vi "Begin.vi"(8 "error in":errorcluster) -> (0 "error out":errorcluster)   [LabVIEW 2016]
doc: "Called before other user functions, this VI is expected to open initial I/O refnums, load in file data, and do all program initialization. Notice that the <B>error out</B> terminal is simply used for data flow. Wiring it to other structures or subVIs ensures that this VI runs first."
uses:
  <vilib>/Rock Robotics/SystemInterfaces/DIO/FPGA_DIOPWMChannel.ctl
  <vilib>/Rock Robotics/WPI/SafetyOutput/WPI_SafetyOutputConfigMenu.ctl
  <vilib>/Rock Robotics/WPI/DriverStation/WPI_DriverStationRobotMode2.ctl
  <vilib>/Rock Robotics/WPI/Joystick/WPI_JoystickDeviceEnum.ctl
  <vilib>/Rock Robotics/SystemInterfaces/DIO/FPGA_DIOChannel.ctl
  <vilib>/Rock Robotics/WPI/Encoder/WPI_EncoderType.ctl
  NI WPI/WPI_SerialPort_USB.ctl
  <vilib>/Rock Robotics/WPI/ThirdParty/CanMotor/TalonSRX/WPI_CANTalonSRX_APIControlMode.ctl
  <vilib>/Rock Robotics/WPI/Solenoid/WPI_SolenoidChannel.ctl
  <vilib>/Rock Robotics/SystemInterfaces/i2clib/i2c_bus.ctl
  Robot Global Data.vi
  <vilib>/Rock Robotics/Network Tables/NT Write String Array.vi
  <vilib>/Rock Robotics/WPI/Counter/WPI_CounterDigitalInputToDigitalSource.vi
  navX Library v2/IO/Open/Z900_navX_Open_Serial.vi
  <vilib>/Rock Robotics/WPI/Solenoid/WPI_SolenoidOpenSingle.vi
  <vilib>/Rock Robotics/WPI/MotorControl/WPI_MotorControlOpen VictorSP.vi
  <vilib>/Rock Robotics/WPI/RobotDrive/WPI_RobotDriveOpen4MotorWithVictorSP.vi
  navX Library v2/navX Library v2.lvlib
  NI WPI/NI WPI Serial USB.lvlib
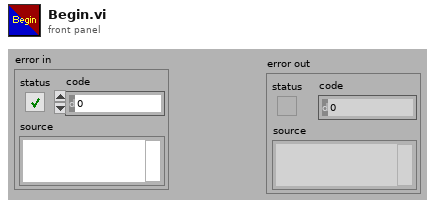
[diagram p1: front panel]
types:
  T1 = typedef "i2c_bus.ctl" = enum16{"I2C On-Board", "I2C MXP", "Invalid"}
  T2 = typedef "WPI_SolenoidChannel.ctl" = enum8{"Solenoid 0", "Solenoid 1", "Solenoid 2", "Solenoid 3", "Solenoid 4", "Solenoid 5", "Solenoid 6", "Solenoid 7", "Invalid"}
  T3 = typedef "FPGA_DIOPWMChannel.ctl" = enum8{"PWM 0", "PWM 1", "PWM 2", "PWM 3", "PWM 4", "PWM 5", "PWM 6", "PWM 7", "PWM 8", "PWM 9", "PWM MXP 0", "PWM MXP 1", "PWM MXP 2", "PWM MXP 3", "PWM MXP 4", "PWM MXP 5", "PWM MXP 6", "PWM MXP 7", "PWM MXP 8", "PWM MXP 9", "Invalid"}
  T4 = typedef "WPI_JoystickDeviceEnum.ctl" = enum16{"USB 0", "USB 1", "USB 2", "USB 3", "USB 4", "USB 5"}
  T5 = typedef "WPI_CANTalonSRX_APIControlMode.ctl" = enum8{"Percent VBus", "Speed", "Position", "Slave", "Unchanged / Invalid", "Voltage Compensation", "Current", "Motion Profile", "Motion Magic"}
  T6 = typedef "NI WPI Serial USB.lvlib/WPI_SerialPort_USB.ctl" = enum16{"Onboard RS-232", "MXP TTL", "USB"}
  T7 = typedef "WPI_EncoderType.ctl" = enum16{"1x", "2x", "4x"}
  T8 = typedef "FPGA_DIOChannel.ctl" = enum8{"DIO 0", "DIO 1", "DIO 2", "DIO 3", "DIO 4", "DIO 5", "DIO 6", "DIO 7", "DIO 8", "DIO 9", "DIO MXP 0", "DIO MXP 1", "DIO MXP 2", "DIO MXP 3", "DIO MXP 4", "DIO MXP 5", "DIO MXP 6", "DIO MXP 7", "DIO MXP 8", "DIO MXP 9", "DIO MXP 10", "DIO MXP 11", "DIO MXP 12", "DIO MXP 13", "DIO MXP 14", "DIO MXP 15", "SPI Port CS1", "SPI Port CS2", "SPI Port CS3", "SPI Port MISO", "SPI Port MOSI", "Invalid"}
  T9 = typedef "WPI_DriverStationRobotMode2.ctl" = enum16{"Autonomous Disabled", "Autonomous Enabled", "Teleop Disabled", "Teleop Enabled", "Disconnected", "Finish", "Test Disabled", "Test Enabled", "Emergency Stopped"}
  T10 = typedef "WPI_SafetyOutputConfigMenu.ctl" = enum16{"Enable", "Disable"}
  T11 = typedef "WPI_JoystickDevRef.ctl" = cluster{"Device":T4}
  T12 = typedef "WPI_I2CDevRef.ctl" = cluster{"DevStatus":errorcluster, "Device Address":u8, "Handle":i32, "I2C Bus":T1}
  T13 = typedef "WPI_MotorControlDeviceRef.ctl" = cluster{"DeviceStatus":errorcluster, "Type":T14, "PWM":cluster{"PWM Channel":T3, "DeadBand":T15}, "CAN":cluster{"Device Number":u8, "SetOutput VI Ref":variant, "GetOutput VI Ref":variant, "Enable VI Ref":variant, "Disable VI Ref":variant, "Data":variant}, "Invert":bool}
  T14 = typedef "WPI_MotorControlType.ctl" = enum16{"PWM", "CAN"}
  T15 = typedef "WPI_PWMDeadband.ctl" = cluster{"Name":string, "maxPositivePwm":i32, "minPositivePwm":i32, "centerPwm":i32, "maxNegativePwm":i32, "minNegativePwm":i32, "angularRange":u16}
  T16 = typedef "WPI_RobotDriveDevRef.ctl" = cluster{"DevStatus":errorcluster, "Motors[]":T13[], "Square Inputs":bool, "Max Output":dbl}
  T17 = typedef "WPI_DigitalInputDevRef.ctl" = cluster{"DevStatus":errorcluster, "DIO Channel":T8}
  T18 = typedef "FPGA_CounterEncoderSourceConvertionLVSourceType.ctl" = cluster{"DevStatus":errorcluster, "AnalogTriggerMode?":bool, "DigitalMode":cluster{"DIO Channel":T19}, "AnalogTriggerMode":cluster{"AnalogTriggerIndex":T20, "OutputType":T21}}
  T19 = typedef "FPGA_DIODigitalSourceChannel.ctl" = enum8{"DIO 0", "DIO 1", "DIO 2", "DIO 3", "DIO 4", "DIO 5", "DIO 6", "DIO 7", "DIO 8", "DIO 9", "DIO MXP 0", "DIO MXP 1", "DIO MXP 2", "DIO MXP 3", "DIO MXP 4", "DIO MXP 5", "DIO MXP 6", "DIO MXP 7", "DIO MXP 8", "DIO MXP 9", "DIO MXP 10", "DIO MXP 11", "DIO MXP 12", "DIO MXP 13", "DIO MXP 14", "DIO MXP 15", "Disabled"}
  T20 = typedef "FPGA_AnalogTriggerIndex.ctl" = enum8{"Trig 0", "Trig 1", "Trig 2", "Trig 3", "Trig 4", "Trig 5", "Trig 6", "Trig 7", "Invalid"}
  T21 = typedef "FPGA_AnalogTriggerOutType.ctl" = enum16{"InWindow", "TriggerState", "Rising", "Falling"}
  T22 = typedef "WPI_EncoderDevRef.ctl" = cluster{"DevStatus":errorcluster, "EncoderIndex":T23, "CounterIndex":T24, "DistancePerCount":dbl, "Decoding Type":T7}
  T23 = typedef "FPGA_EncoderIdx.ctl" = enum8{"Enc 0", "Enc 1", "Enc 2", "Enc 3", "Enc 4", "Enc 5", "Enc 6", "Enc 7", "Invalid"}
  T24 = typedef "FPGA_CounterCtrSystemIndex.ctl" = enum8{"Ctr 0", "Ctr 1", "Ctr 2", "Ctr 3", "Ctr 4", "Ctr 5", "Ctr 6", "Ctr 7", "Invalid"}
  T25 = typedef "navX Library v2.lvlib/Z900_navX_DeviceTypeDef.ctl" = cluster{"Interface":cluster{"Protocol":T26, "Update Rate (4Hz-100Hz)":u8, "navX Open TypeDef":variant}, "Notify Packet":refnum<notifier>, "Loop VI Refnum":refnum<vi>, "Ready to Close Occurrence Refnum":refnum<k4>}
  T26 = typedef "navX Library v2.lvlib/Z900_navX_ProtocolTypeDef.ctl" = enum16{"SERIAL", "I2C", "SPI"}
  T27 = typedef "WPI_SolenoidDevRef.ctl" = cluster{"DevStatus":errorcluster, "Pneumatics Control Module":u8, "Forward Solenoid Channel":T2, "Reverse Solenoid Channel":T2}
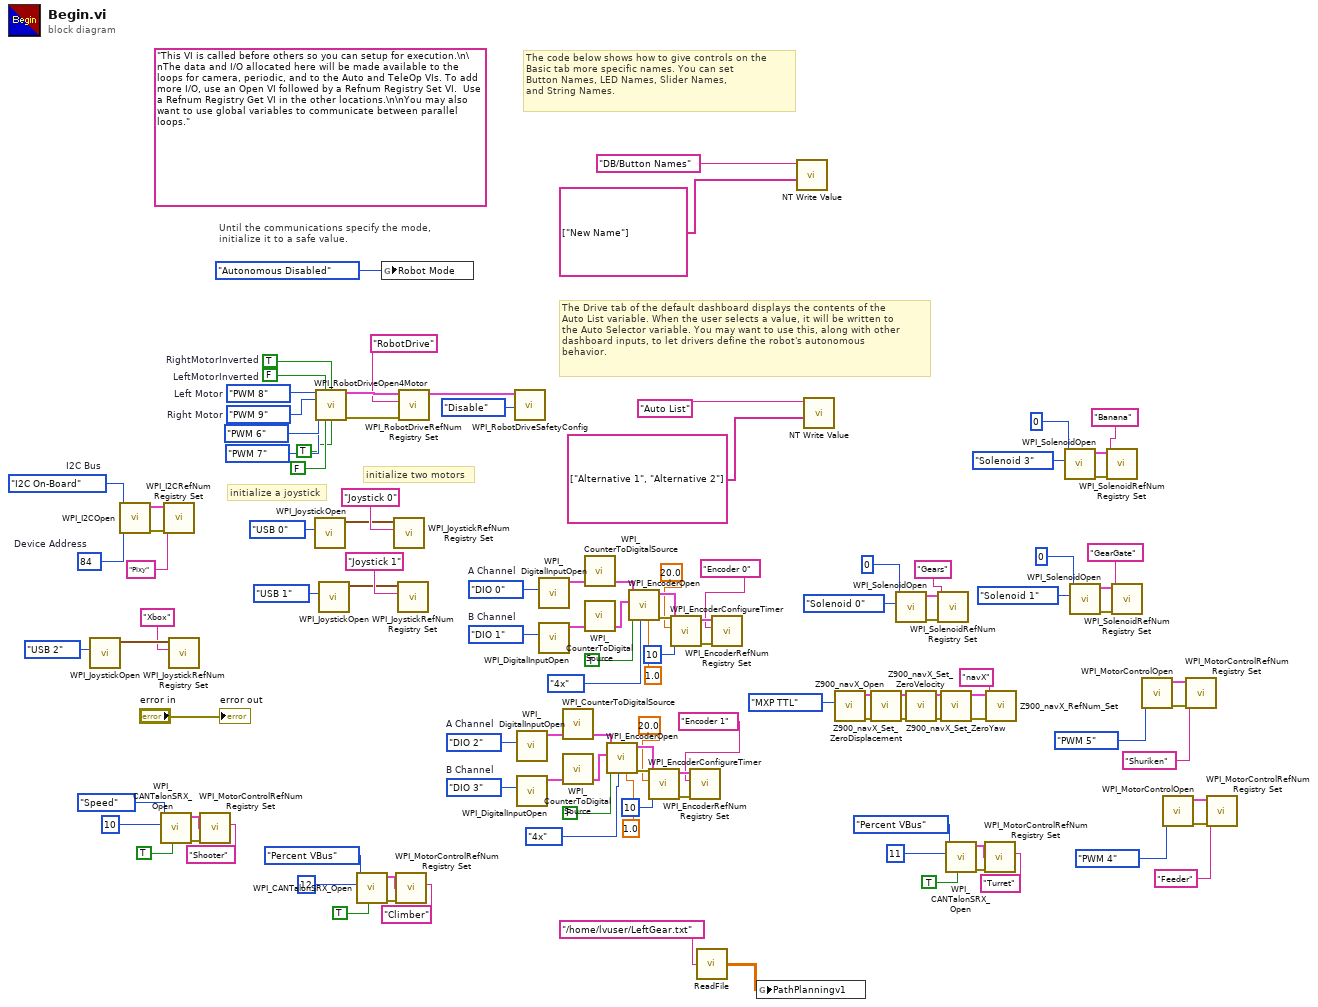
[diagram p0: block diagram]
diagram:
  w8 = u8 84  # Device Address
  w9 = i2c_bus."I2C On-Board"  # I2C Bus
  w81 = FPGA_DIOChannel."DIO 3"  # B Channel
  w80 = FPGA_DIOChannel."DIO 2"  # A Channel
  w97 = FPGA_DIOChannel."DIO 1"  # B Channel
  w96 = FPGA_DIOChannel."DIO 0"  # A Channel
  (unwired) "This VI is called before others so you can setup for execution.\n\nThe data and I/O allocated here will be made available to the loops for camera, periodic, and to the Auto and TeleOp VIs. To add more I/O, use an Open VI followed by a Refnum Registry Set VI.  Use a Refnum Registry Get VI in the other locations.\n\nYou may also want to use global variables to communicate between parallel loops."
  w112 = FPGA_DIOPWMChannel."PWM 9"  # Right Motor
  w113 = FPGA_DIOPWMChannel."PWM 8"  # Left Motor
  w117 = FALSE  # LeftMotorInverted
  w118 = TRUE  # RightMotorInverted
  # "The Drive tab of the default dashboard displays the contents of the\nAuto List variable. When the user selects a value, it will be written to\nthe Auto Selector variable. You may want to use this, along with other\ndashboard inputs, to let drivers define the robot's autonomous\nbehavior."
  # "The code below shows how to give controls on the\nBasic tab more specific names. You can set\nButton Names, LED Names, Slider Names,\nand String Names."
  # "initialize a joystick"
  # "Until the communications specify the mode,\ninitialize it to a safe value."
  # "initialize two motors"
  n1 = call <vilib>:"WPI_JoystickOpen.vi"("JoystickDevice"=WPI_JoystickDeviceEnum."USB 2") -> ("JoystickDevRef"=w21:T11)  [unwired: 10 in]
  n2 = call <vilib>:"WPI_I2COpen.vi"("Device Address"=w8, "I2C Bus"=w9) -> ("error out"=w7:errorcluster, "I2CDevRef"=w6:T12)  [unwired: 8 in]
  n3 = call <vilib>:"WPI_CANTalonSRX_Open.vi"("Invert"=TRUE, "Device Number"=10, "Control Mode"=WPI_CANTalonSRX_APIControlMode."Speed") -> ("error out"=w48:errorcluster, "CAN Talon SRX Ref"=w49:T13)  [unwired: 7 in]
  n4 = call <vilib>:"WPI_I2CRefNum Registry Set.vi"("error in (no error)"=w7, "refnum name"="Pixy", "I2CDevRef"=w6) -> ()  [unwired: 7 in, 2 out]
  n5 = call <vilib>:"WPI_JoystickRefNum Registry Set.vi"("refnum name"="Xbox", "JoystickDevRef"=w21) -> ()  [unwired: 8 in, 2 out]
  n6 = call <vilib>:"WPI_MotorControlRefNum Registry Set.vi"("error in (no error)"=w48, "refnum name"="Shooter", "MotorControlDevRef"=w49) -> ()  [unwired: 7 in, 2 out]
  n7 = call <vilib>:"WPI_JoystickOpen.vi"("JoystickDevice"=WPI_JoystickDeviceEnum."USB 0") -> ("JoystickDevRef"=w107:T11)  [unwired: 10 in]
  n8 = call-poly <vilib>:"WPI_RobotDriveOpen4Motor.vi"("Rear Left Motor"=w113, "Rear Left Motor Inverted"=w117, "Rear Right Motor Inverted"=w118, "Rear Right Motor"=w112, "Front Left Motor"=FPGA_DIOPWMChannel."PWM 6", "Front Right Motor"=FPGA_DIOPWMChannel."PWM 7", "Front Left Motor Inverted"=FALSE, "Front Right Motor Inverted"=TRUE) -> ("RobotDriveDevRef"=w116:T16, "error out"=w114:errorcluster)  [unwired: 6 in]
  n9 = call <vilib>:"WPI_JoystickOpen.vi"("JoystickDevice"=WPI_JoystickDeviceEnum."USB 1") -> ("JoystickDevRef"=w99:T11)  [unwired: 10 in]
  n10 = call <vilib>:"WPI_CANTalonSRX_Open.vi"("Invert"=TRUE, "Device Number"=12, "Control Mode"=WPI_CANTalonSRX_APIControlMode."Percent VBus") -> ("error out"=w42:errorcluster, "CAN Talon SRX Ref"=w43:T13)  [unwired: 7 in]
  n11 = global write "Robot Global Data.vi" "Robot Mode"(WPI_DriverStationRobotMode2."Autonomous Disabled" ("Robot Mode")) -> ()
  n12 = call <vilib>:"WPI_JoystickRefNum Registry Set.vi"("refnum name"="Joystick 0", "JoystickDevRef"=w107) -> ()  [unwired: 8 in, 2 out]
  n13 = call <vilib>:"WPI_MotorControlRefNum Registry Set.vi"("error in (no error)"=w42, "refnum name"="Climber", "MotorControlDevRef"=w43) -> ()  [unwired: 7 in, 2 out]
  n14 = call <vilib>:"WPI_JoystickRefNum Registry Set.vi"("refnum name"="Joystick 1", "JoystickDevRef"=w99) -> ()  [unwired: 8 in, 2 out]
  n15 = call <vilib>:"WPI_RobotDriveRefNum Registry Set.vi"("error in (no error)"=w114, "refnum name"="RobotDrive", "RobotDriveDevRef"=w116) -> ("RobotDriveDevRef"=w111:T16)  [unwired: 1 in, 7 out]
  n16 = call <vilib>:"WPI_RobotDriveSafetyConfig.vi"("mode"=WPI_SafetyOutputConfigMenu."Disable", "RobotDriveDevRef"=w111) -> ()  [unwired: 8 in, 2 out]
  n17 = call <vilib>:"WPI_DigitalInputOpen.vi"("DIO Channel"=w80) -> ("DigitalInputDevRef"=w77:T17)  [unwired: 1 in, 9 out]
  n18 = call <vilib>:"WPI_DigitalInputOpen.vi"("DIO Channel"=w81) -> ("DigitalInputDevRef"=w78:T17)  [unwired: 1 in, 9 out]
  n19 = call <vilib>:"WPI_DigitalInputOpen.vi"("DIO Channel"=w96) -> ("DigitalInputDevRef"=w93:T17)  [unwired: 1 in, 9 out]
  n20 = call <vilib>:"WPI_DigitalInputOpen.vi"("DIO Channel"=w97) -> ("DigitalInputDevRef"=w94:T17)  [unwired: 1 in, 9 out]
  n21 = call-poly <vilib>:"WPI_CounterToDigitalSource.vi"("DigitalInputDevRef"=w77) -> ("Digital Source"=w76:T18)  [unwired: 6 out]
  n22 = call-poly <vilib>:"WPI_CounterToDigitalSource.vi"("DigitalInputDevRef"=w78) -> ("Digital Source"=w79:T18)  [unwired: 6 out]
  n23 = call-poly <vilib>:"WPI_CounterToDigitalSource.vi"("DigitalInputDevRef"=w93) -> ("Digital Source"=w92:T18)  [unwired: 6 out]
  n24 = call-poly <vilib>:"WPI_CounterToDigitalSource.vi"("DigitalInputDevRef"=w94) -> ("Digital Source"=w95:T18)  [unwired: 6 out]
  n25 = call <vilib>:"WPI_EncoderOpen.vi"("DistancePerCount"=1.0, "Decoding Type"=WPI_EncoderType."4x", "Invert Direction (False)"=FALSE, "BSource"=w79, "ASource"=w76) -> ("error out"=w74:errorcluster, "EncoderDevRef"=w73:T22)  [unwired: 3 in, 2 out]
  n26 = call <vilib>:"WPI_EncoderOpen.vi"("DistancePerCount"=1.0, "Decoding Type"=WPI_EncoderType."4x", "Invert Direction (False)"=TRUE, "BSource"=w95, "ASource"=w92) -> ("error out"=w88:errorcluster, "EncoderDevRef"=w87:T22)  [unwired: 3 in, 2 out]
  n27 = call <vilib>:"WPI_EncoderConfigureTimer.vi"("error in (no error)"=w74, "Number Samples to Average"=u8 10, "Minimum Rate"=20.0, "EncoderDevRef"=w73) -> ("error out"=w70:errorcluster, "EncoderDevRef"=w69:T22)  [unwired: 6 in]
  n28 = call <vilib>:"WPI_EncoderConfigureTimer.vi"("error in (no error)"=w88, "Number Samples to Average"=u8 10, "Minimum Rate"=20.0, "EncoderDevRef"=w87) -> ("error out"=w84:errorcluster, "EncoderDevRef"=w83:T22)  [unwired: 6 in]
  n29 = call <vilib>:"WPI_EncoderRefNum Registry Set.vi"("error in (no error)"=w70, "refnum name"="Encoder 1", "EncoderDevRef"=w69) -> ()  [unwired: 7 in, 2 out]
  n30 = call "ReadFile.vi"("Name"="/home/lvuser/LeftGear.txt") -> ("Array - Numeric"=w3:dbl[][])
  n31 = call <vilib>:"WPI_EncoderRefNum Registry Set.vi"("error in (no error)"=w84, "refnum name"="Encoder 0", "EncoderDevRef"=w83) -> ()  [unwired: 7 in, 2 out]
  n32 = global write "Robot Global Data.vi" "PathPlanningv1"(w3) -> ()
  n33 = call-poly <vilib>:"NT Write Value.vi"("String Array"=string[] ["New Name"], "Name"="DB/Button Names") -> ()  [unwired: 9 in, 1 out]
  n34 = call-poly <vilib>:"NT Write Value.vi"("String Array"=string[] ["Alternative 1", "Alternative 2"], "Name"="Auto List") -> ()  [unwired: 9 in, 1 out]
  n35 = call-poly "Z900_navX_Open.vi"("Serial Port"=WPI_SerialPort_USB."MXP TTL") -> ("error out"=w56:errorcluster, "navX Device"=w61:T25)  [unwired: 9 in]
  n36 = call "Z900_navX_Set_ZeroDisplacement.vi"("error in (no error)"=w56, "navX Device"=w61) -> ("error out"=w55:errorcluster, "navX Device"=w60:T25)  [unwired: 8 in]
  n37 = call-poly <vilib>:"WPI_SolenoidOpen.vi"("Solenoid Channel"=WPI_SolenoidChannel."Solenoid 0", "Pneumatics Control Module (0)"=u8 0) -> ("error out"=w41:errorcluster, "SolenoidDevRef"=w40:T27)  [unwired: 8 in]
  n38 = call "Z900_navX_Set_ZeroVelocity.vi"("error in (no error)"=w55, "navX Device"=w60) -> ("error out"=w54:errorcluster, "navX Device"=w59:T25)  [unwired: 8 in]
  n39 = call <vilib>:"WPI_SolenoidRefNum Registry Set.vi"("error in (no error)"=w41, "refnum name"="Gears", "SolenoidDevRef"=w40) -> ()  [unwired: 7 in, 2 out]
  n40 = call "Z900_navX_Set_ZeroYaw.vi"("error in (no error)"=w54, "navX Device"=w59) -> ("error out"=w57:errorcluster, "navX Device"=w58:T25)  [unwired: 8 in]
  n41 = call <vilib>:"WPI_CANTalonSRX_Open.vi"("Invert"=TRUE, "Device Number"=11, "Control Mode"=WPI_CANTalonSRX_APIControlMode."Percent VBus") -> ("error out"=w31:errorcluster, "CAN Talon SRX Ref"=w32:T13)  [unwired: 7 in]
  n42 = call <vilib>:"WPI_MotorControlRefNum Registry Set.vi"("error in (no error)"=w31, "refnum name"="Turret", "MotorControlDevRef"=w32) -> ()  [unwired: 7 in, 2 out]
  n43 = call "Z900_navX_RefNum_Set.vi"("error in (no error)"=w57, "refnum name"="navX", "navX Device"=w58) -> ()  [unwired: 7 in, 2 out]
  n44 = call-poly <vilib>:"WPI_SolenoidOpen.vi"("Solenoid Channel"=WPI_SolenoidChannel."Solenoid 3", "Pneumatics Control Module (0)"=u8 0) -> ("error out"=w14:errorcluster, "SolenoidDevRef"=w13:T27)  [unwired: 8 in]
  n45 = call-poly <vilib>:"WPI_SolenoidOpen.vi"("Solenoid Channel"=WPI_SolenoidChannel."Solenoid 1", "Pneumatics Control Module (0)"=u8 0) -> ("error out"=w26:errorcluster, "SolenoidDevRef"=w25:T27)  [unwired: 8 in]
  n46 = call <vilib>:"WPI_SolenoidRefNum Registry Set.vi"("error in (no error)"=w14, "refnum name"="Banana", "SolenoidDevRef"=w13) -> ()  [unwired: 7 in, 2 out]
  n47 = call <vilib>:"WPI_SolenoidRefNum Registry Set.vi"("error in (no error)"=w26, "refnum name"="GearGate", "SolenoidDevRef"=w25) -> ()  [unwired: 7 in, 2 out]
  n48 = call-poly <vilib>:"WPI_MotorControlOpen.vi"("PWM Channel"=FPGA_DIOPWMChannel."PWM 5") -> ("error out"=w30:errorcluster, "MotorControlDeviceRef"=w29:T13)  [unwired: 9 in]
  n49 = call-poly <vilib>:"WPI_MotorControlOpen.vi"("PWM Channel"=FPGA_DIOPWMChannel."PWM 4") -> ("error out"=w18:errorcluster, "MotorControlDeviceRef"=w17:T13)  [unwired: 9 in]
  n50 = call <vilib>:"WPI_MotorControlRefNum Registry Set.vi"("error in (no error)"=w30, "refnum name"="Shuriken", "MotorControlDevRef"=w29) -> ()  [unwired: 7 in, 2 out]
  n51 = call <vilib>:"WPI_MotorControlRefNum Registry Set.vi"("error in (no error)"=w18, "refnum name"="Feeder", "MotorControlDevRef"=w17) -> ()  [unwired: 7 in, 2 out]
  "error out" <- "error in"
